vi "HexToNormal.vi"(11 "String in":string) -> (3 "String Out":string)   [LabVIEW 2013, in "main.lvlib"]
uses:
  main.lvlib
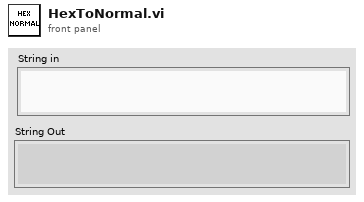
[diagram p1: front panel]
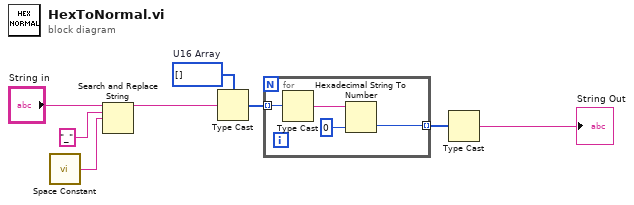
[diagram p0: block diagram]
diagram:
  w8 = u16[] []  # U16 Array
  n1 = call <vilib>:"Space Constant.vi"() -> ("String"=w1:string)
  n2 = Search and Replace String(input string="String in", search string="_", replace string=w1) -> (result string=w3:string)  [unwired: 5 in, 3 out]
  n3 = Type Cast(type=w8, x=w3) -> (*(type *) &x=w7:u16[])
  n4 = for {
    tunnel: w7 -> [w12] mode=indexing
    tunnel: [w9] -> w6 mode=indexing
    n5 = Type Cast(x=w12) -> (*(type *) &x=w11:string)  [unwired: 1 in]
    n6 = Hexadecimal String To Number(string=w11, default (0uL)=u8 0) -> (number=w9:u8)  [unwired: 1 in, 1 out]
  }
  n7 = Type Cast(x=w6) -> (*(type *) &x=→"String Out":string)  [unwired: 1 in]
